vi "WPI_GetFilterFrequency.vi"(8 "error in (no error)":errorcluster, 11 "DigitalInputDevRef":T1={"DevStatus"={"status"=FALSE, "code"=0, "source"=""}, "DIO Channel"=enum."DIO 1"}) -> (0 "error out":errorcluster, 1 "Filter Enabled":bool, 2 "Filter Frequency":dbl=76628.35249042146, 3 "DigitalInputDevRef":T1={"DevStatus"={"status"=FALSE, "code"=0, "source"=""}, "DIO Channel"=enum."DIO 1"})   [LabVIEW 2017]
doc: "Returns whether a digital input filter is enabled and the frequency of the filter.\n\nThis software is licensed. Open the labview\\readme\\WPI Robotics Library Open Source License.txt file for more information."
uses:
  <vilib>/Rock Robotics/WPI/DigitalInput/WPI_DigitalInputDevRef.ctl
  <vilib>/Rock Robotics/SystemInterfaces/DIO/FPGA_DIOChannel.ctl
  <vilib>/Rock Robotics/SystemInterfaces/System/FPGA_SystemGet.vi
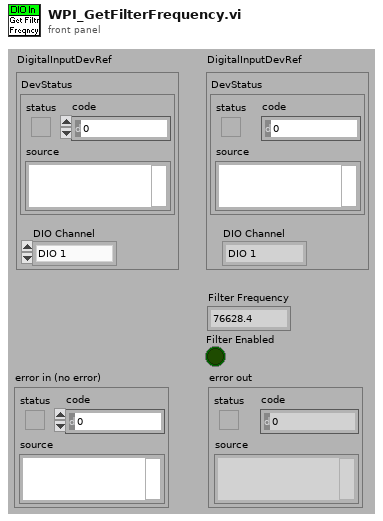
[diagram p1: front panel]
types:
  T1 = typedef "WPI_DigitalInputDevRef.ctl" = cluster{"DevStatus":errorcluster, "DIO Channel":T2}
  T2 = typedef "FPGA_DIOChannel.ctl" = enum8{"DIO 0", "DIO 1", "DIO 2", "DIO 3", "DIO 4", "DIO 5", "DIO 6", "DIO 7", "DIO 8", "DIO 9", "DIO MXP 0", "DIO MXP 1", "DIO MXP 2", "DIO MXP 3", "DIO MXP 4", "DIO MXP 5", "DIO MXP 6", "DIO MXP 7", "DIO MXP 8", "DIO MXP 9", "DIO MXP 10", "DIO MXP 11", "DIO MXP 12", "DIO MXP 13", "DIO MXP 14", "DIO MXP 15", "SPI Port CS1", "SPI Port CS2", "SPI Port CS3", "SPI Port MISO", "SPI Port MOSI", "Invalid"}
  T3 = typedef "FPGA_DIODevRef.ctl" = cluster{"DevStatus":errorcluster}
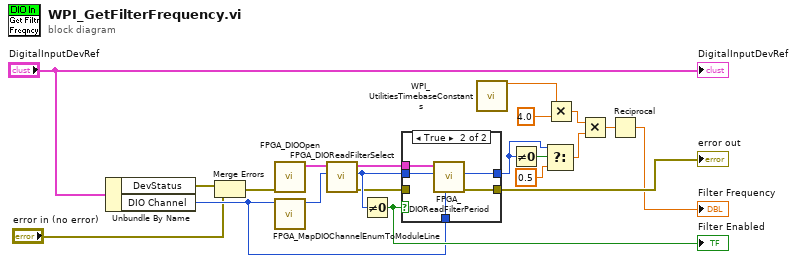
[diagram p0: block diagram]
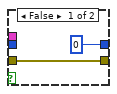
[diagram p2: hidden frame]
diagram:
  n1 = Unbundle By Name("DigitalInputDevRef") -> ("DevStatus"=w6:errorcluster, "DIO Channel"=w4:T2)
  n2 = Merge Errors(w6, "error in (no error)") -> (w5:errorcluster)
  n3 = call <vilib>:"FPGA_DIOOpen.vi"("error in (no error)"=w5) -> ("DIODeviceRef"=w18:T3)  [unwired: 1 in, 9 out]
  n4 = call <vilib>:"FPGA_MapDIOChannelEnumToModuleLine.vi"("DIOChannel"=w4) -> ("ActualDIOChannel(U8)"=w17:u8)  [unwired: 10 out]
  n5 = call <vilib>:"FPGA_DIOReadFilterSelect.vi"("channel index"=w17, "DIODeviceRef In"=w18) -> ("error out"=w14:errorcluster, "FilterSelect"=w15:u8, "DIODeviceRef Out"=w16:T3)  [unwired: 1 in, 6 out]
  n6 = Not Equal To 0?(x=w15) -> (x != 0?=w20:bool)
  "Filter Enabled" <- w20
  n7 = case shown="True" w20 {
    tunnel: w16 -> [_ w28]
    tunnel: w15 -> [_ w25]
    tunnel: [u8 0 ("PWMFilterPeriod") w27] -> w10
    tunnel: w14 -> [w22 _]
    tunnel: [w22 w26] -> w21
    tunnel: w4 -> [_ w24]
    frame False {
    }
    frame True {
      n8 = call <vilib>:"FPGA_DIOReadFilterPeriod.vi"("DIOChannel"=w24, "index"=w25, "DIODeviceRef In"=w28) -> ("error out"=w26:errorcluster, "PWMFilterPeriod"=w27:u32)  [unwired: 1 in, 6 out]
    }
  }
  "error out" <- w21
  n9 = call <vilib>:"WPI_UtilitiesTimebaseConstants.vi"() -> ("40 MHz FPGA clock"=w3:dbl)  [unwired: 13 in, 2 out]
  n10 = Not Equal To 0?(x=w10) -> (x != 0?=w11:bool)
  n11 = Select(t=w10, s=w11, f=0.5) -> (s? t:f=w8:dbl)
  n12 = Multiply(x=w3, y=4.0) -> (x*y=w13:dbl)
  n13 = Multiply(x=w13, y=w8) -> (x*y=w7:dbl)
  n14 = Reciprocal(x=w7) -> (1/x=→"Filter Frequency":dbl)
  "DigitalInputDevRef" <- "DigitalInputDevRef"
